vi "WaterTankExample.vi"() -> ()   [LabVIEW 2017, in "Examples.lvlib"]
uses:
  Examples.lvlib
panel:
  in  "Stop Button":bool
  in  "Drainage (litres/s)":dbl(slide) scale=0.0..10.0
  in  "Flow in (litres/s)":dbl(slide) scale=0.0..10.0
  out "Indicator":bool
  out "Indicator":bool
  out "Tank (litres)":dbl(slide) scale=0.0..100.0
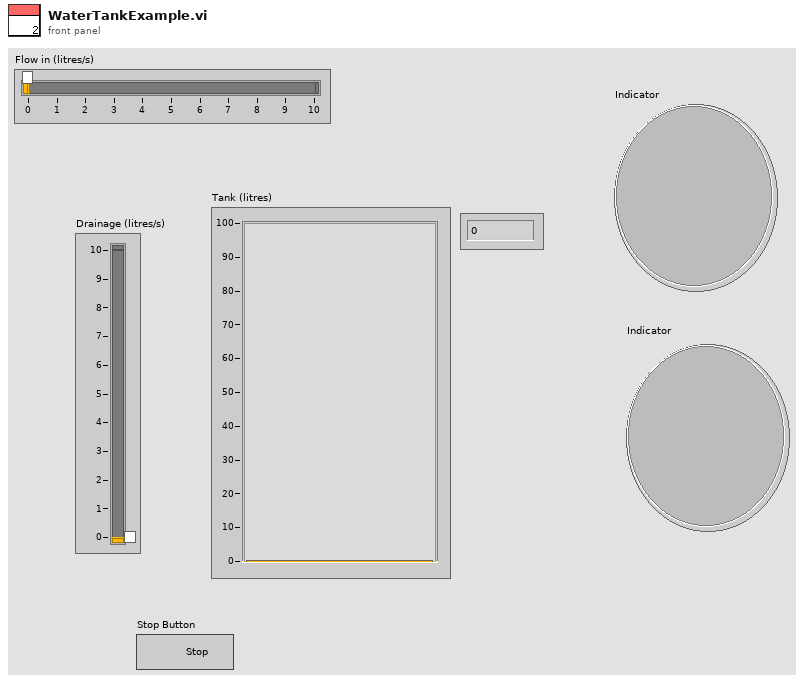
[diagram p1: front panel]
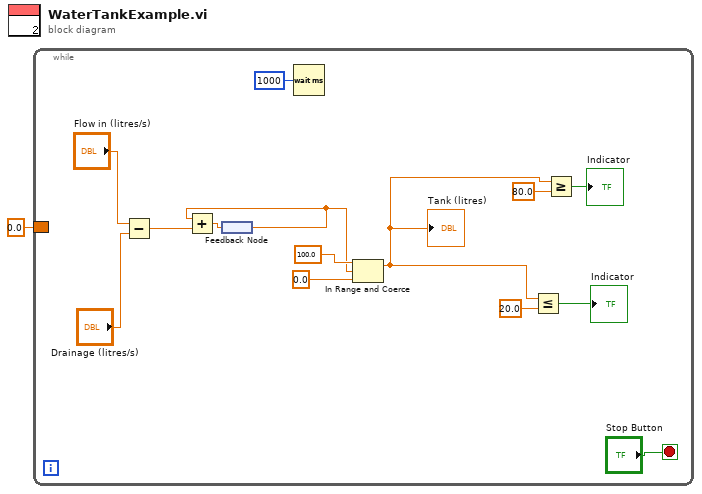
[diagram p0: block diagram]
diagram:
  n1 = while {
    border: 0.0 -> [_]
    stop <- "Stop Button" stop-if-true
    n2 = Subtract(x="Flow in (litres/s)", y="Drainage (litres/s)") -> (x-y=w12:dbl)
    n3 = feedback #1() -> (w7:dbl)
    n4 = Add(x=w7, y=w12) -> (x+y=w10:dbl)
    n5 = feedback-in #1(w10) -> ()
    n6 = Wait (ms)(milliseconds to wait=u32 1000) -> ()  [unwired: 1 out]
    n7 = In Range and Coerce(upper limit=100.0, x=w7, lower limit=0.0) -> (coerced(x)=w2:dbl)  [unwired: 1 out]
    "Tank (litres)" <- w2
    n8 = Less Or Equal?(x=w2, y=20.0) -> (x <= y?=→"Indicator":bool)
    n9 = Greater Or Equal?(x=w2, y=80.0) -> (x >= y?=→"Indicator":bool)
  }
